vi "readDAQwaveform.vi"(0 "channel (0)":tag="0") -> (1 "channel out":tag="0", 2 "Waveform Graph":waveform(dbl)(graph), 3 "Waveform Cluster":cluster{"t0":timestamp, "dt":dbl, "Y":dbl[]} {"Y" format="%0.2f"; "dt" format="%0.2f"; "t0" format="%<%X\n%x>T"}, 4 "error out":errorcluster)   [LabVIEW 2013]
uses:
  <vilib>/Daq/Ai.llb/AI Waveform Scan (waveform).vi
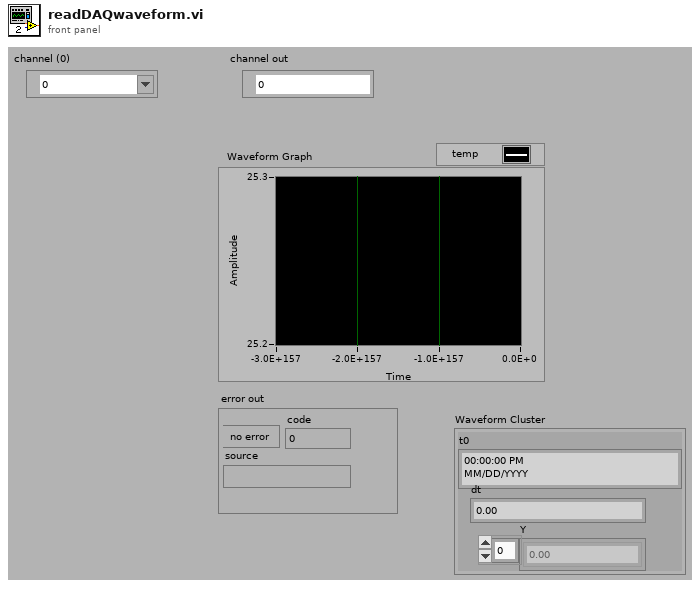
[diagram p1: front panel]
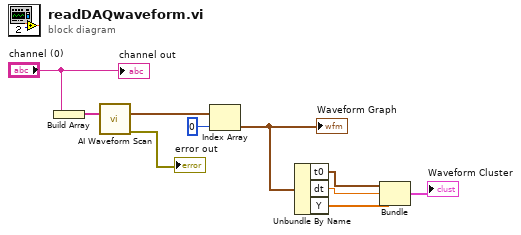
[diagram p0: block diagram]
diagram:
  n1 = Build Array("channel (0)") -> (w9:tag[])
  n2 = call-poly <vilib>:"AI Waveform Scan.vi"("channels (0)"=w9) -> ("waveform data"=w7:waveform(dbl)[], "error out"=→"error out":errorcluster)  [unwired: 7 in, 6 out]
  n3 = Index Array(array=w7, index=0 ("Index")) -> (element=w1:waveform(dbl))
  "Waveform Graph" <- w1
  n4 = Unbundle By Name(w1) -> ("t0"=w5:timestamp, "dt"=w4:dbl, "Y"=w3:dbl[])
  n5 = Bundle("t0"=w5, "dt"=w4, "Y"=w3) -> (→"Waveform Cluster":cluster{"t0":timestamp, "dt":dbl, "Y":dbl[]})  [unwired: 1 out]
  "channel out" <- "channel (0)"
